vi "sv_Correct Optimal Transition Time.vi"(10 "dt":dbl, 11 "time to optimum [s]":dbl) -> (3 "corrected time to optimum [s]":dbl)   [LabVIEW 2017, in "SoundVib_Generation.lvlib"]
uses:
  <vilib>/addons/_NISVFA/_Generation/SoundVib_Generation.lvlib
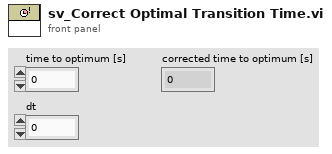
[diagram p1: front panel]
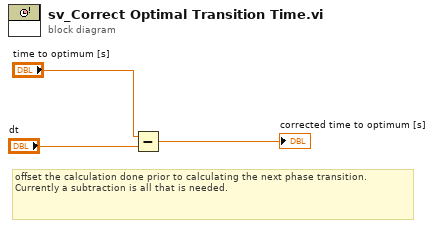
[diagram p0: block diagram]
diagram:
  # "offset the calculation done prior to calculating the next phase transition. Currently a subtraction is all that is needed."
  n1 = Subtract(x="time to optimum [s]", y="dt") -> (x-y=→"corrected time to optimum [s]":dbl)
